vi "Soy_Create.vi"(0 "reference in":refnum<class "Soy.lvclass">, 2 "Beverage":refnum<class "Beverage.lvclass">, 5 "error in (no error)":errorcluster) -> (14 "reference out":refnum<class "Soy.lvclass">, 19 "error out":errorcluster)   [LabVIEW 2020, in "Soy.lvclass"]
uses:
  Soy.lvclass
  C:/Projects/OpenGDS_DesignPatterns/Decorator1/CondimentDecorator_class/CondimentDecorator.lvclass
  Beverage_class/Beverage.lvclass
  CondimentDecorator_class/CondimentDecorator.lvclass
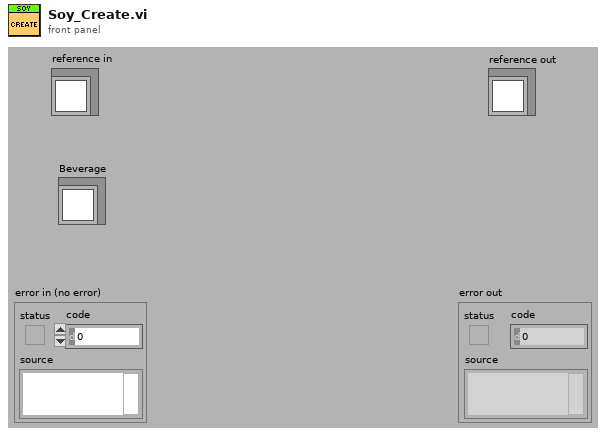
[diagram p1: front panel]
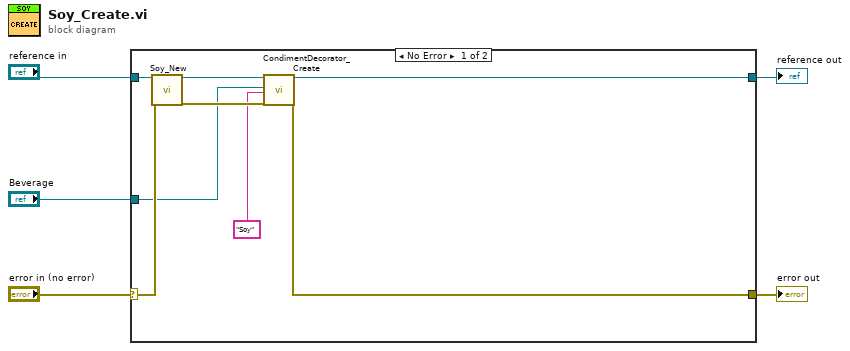
[diagram p0: block diagram]
diagram:
  n1 = case shown="No Error" "error in (no error)" {
    selector: "error in (no error)" -> [w12 w15]
    tunnel: [w6 w15] -> w4
    tunnel: "reference in" -> [w13 w14]
    tunnel: [w9 w14] -> w2
    tunnel: "Beverage" -> [w8 _]
    frame No Error {
      n2 = call "Soy_New.vi"("reference in"=w13, "error in (no error)"=w12) -> ("reference out"=w11:refnum<class "Soy.lvclass">, "error out"=w10:errorcluster)  [unwired: 14 in, 2 out]
      n3 = call "CondimentDecorator_Create.vi"("reference in"=w11, "Beverage"=w8, "CondimentName"="Soy", "error in (no error)"=w10) -> ("reference out"=w9:refnum<class "Soy.lvclass">, "error out"=w6:errorcluster)  [unwired: 14 in]
    }
    frame Error {
    }
  }
  "error out" <- w4
  "reference out" <- w2
